vi "读取CODMn数据波形新.vi"() -> ()   [LabVIEW 2016, in "斯坦道CODMn.lvlib"]
uses:
  <vilib>/Utility/miscctls.llb/LVPointTypeDef.ctl
  <userlib>/_OpenG.lib/array/array.llb/Sort 1D Array (I32)__ogtk.vi
  <vilib>/Waveform/WDTFileIO.llb/Read Waveform from File.vi
panel:
  in  "页":i32 format="第%.0f页"
  in  "每页条数":i32=20
  in  "向后按钮":bool
  in  "向前按钮":bool
  in  "数据表":T1
  in  "查看曲线数组":bool[](array[boolean])
  in  "打开波形文件":bool
  in  "簇":cluster{"数据起始时间":timestamp, "数据终止时间":timestamp}
  in  "查询":bool
  in  "当前滴定曲线":bool
  in  "当前温度曲线":bool
  in  "关闭":bool
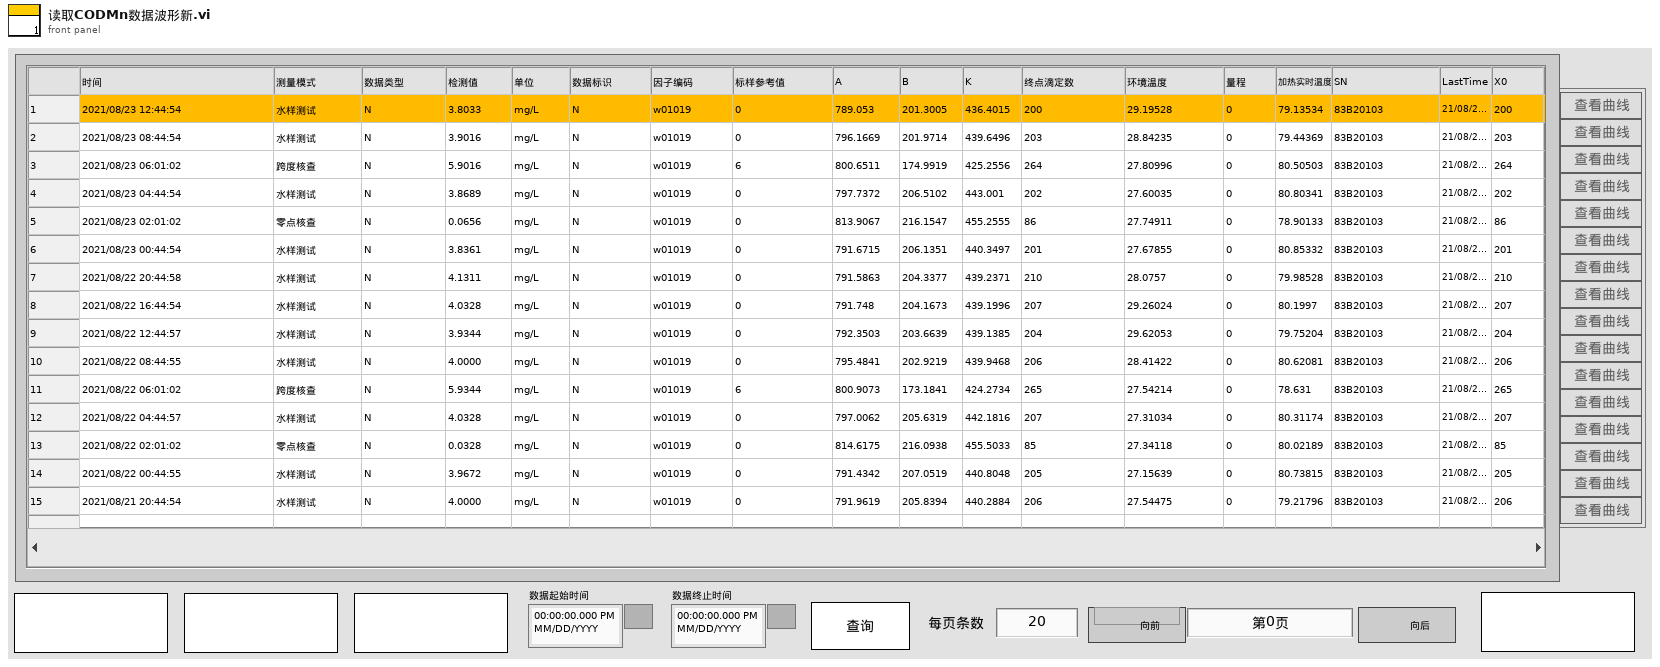
[diagram p1: front panel]
types:
  T1 = typedef "斯坦道CODMn.lvlib/数据查询大列表框.ctl" = i32
  T2 = typedef "LVPointTypeDef.ctl" = cluster{"Horizontal":i16, "Vertical":i16}
  T3 = cluster{timestamp, "seconds since 1Jan1904":timestamp}
  T4 = enum16{"Left Button", "Center Button", "Right Button", "Window Close"}
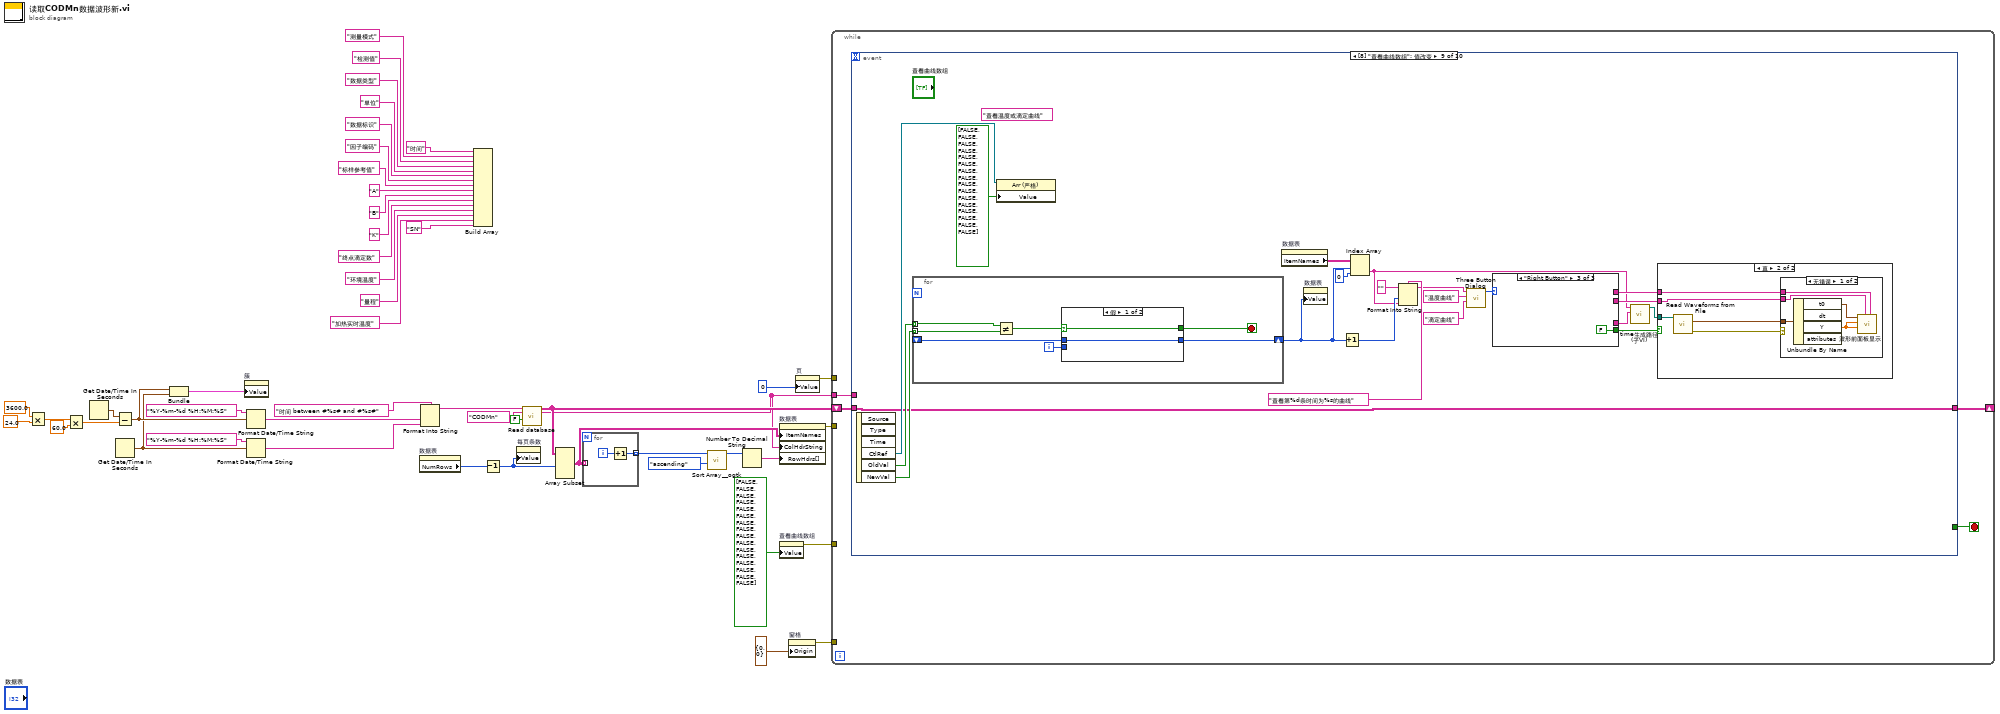
[diagram p0: block diagram]
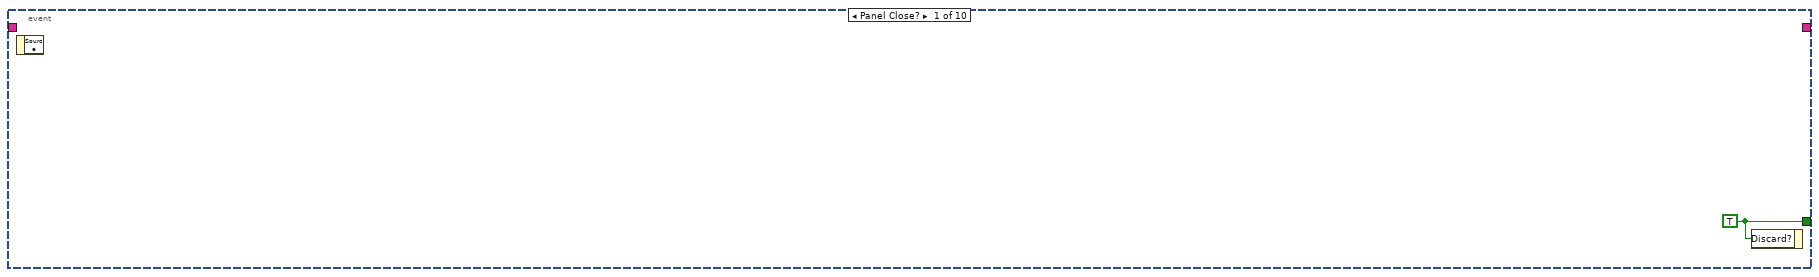
[diagram p2: hidden frame]
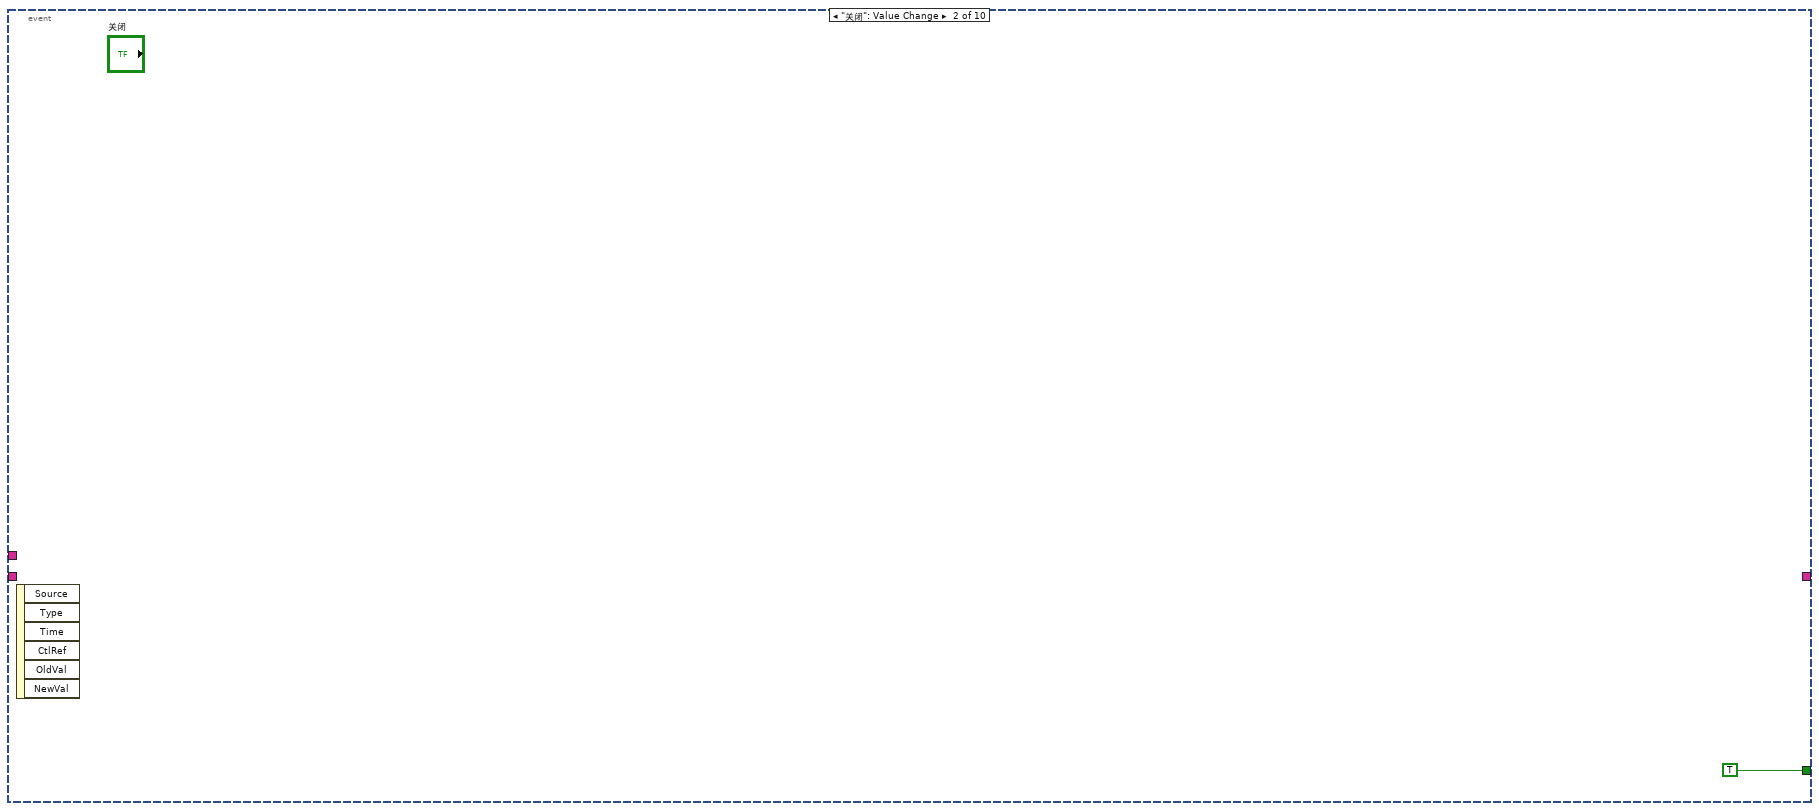
[diagram p3: hidden frame]
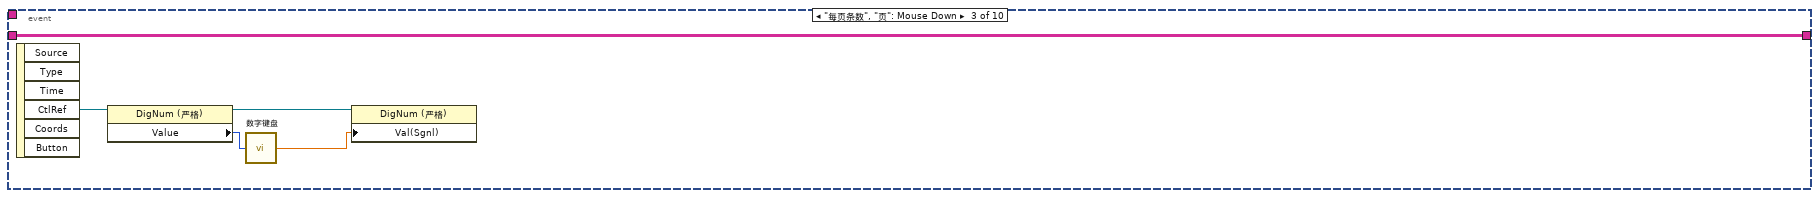
[diagram p4: hidden frame]
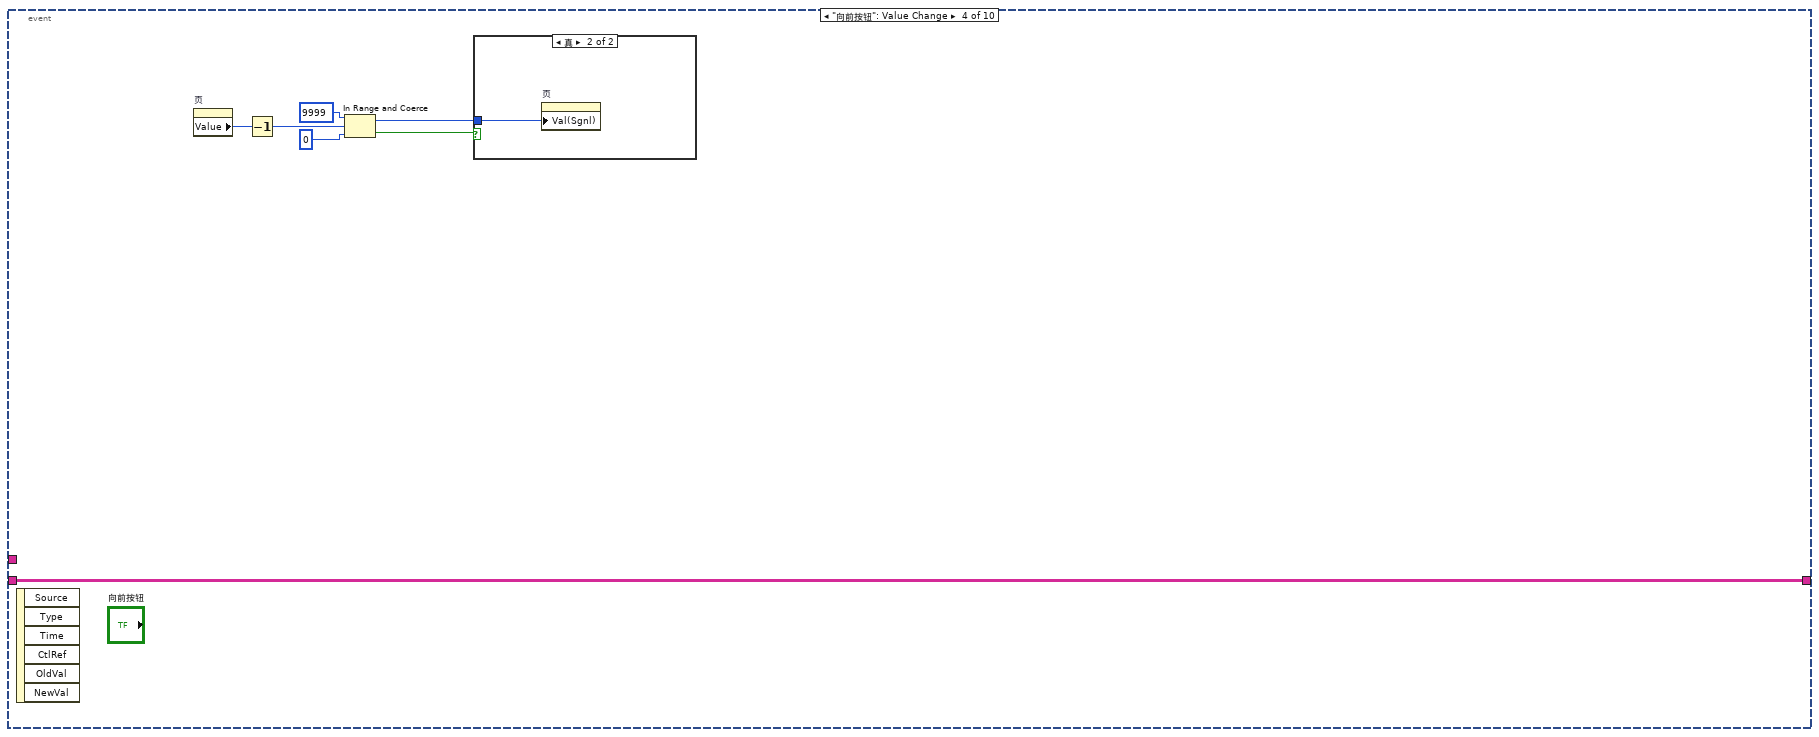
[diagram p5: hidden frame]
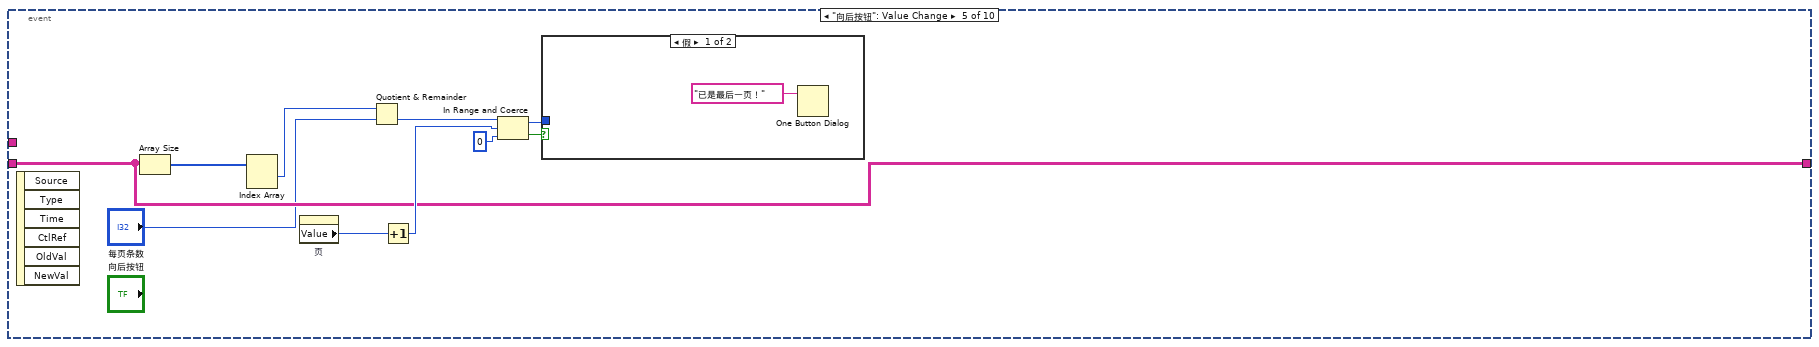
[diagram p7: hidden frame]
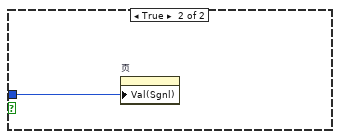
[diagram p8: hidden frame]
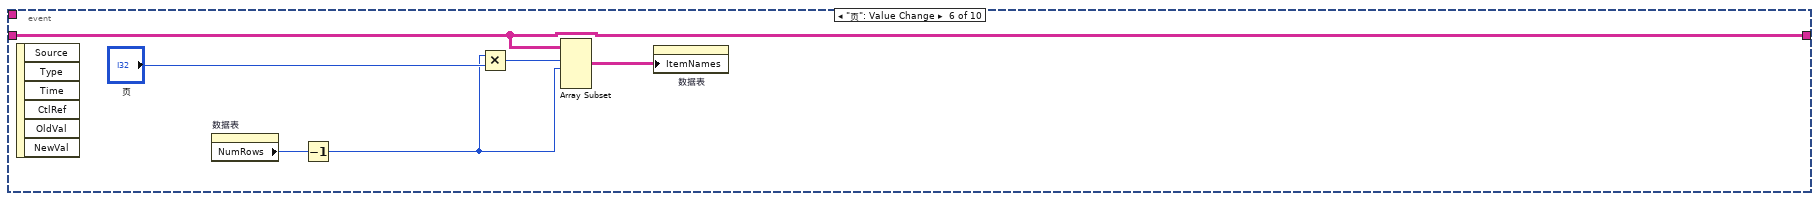
[diagram p9: hidden frame]
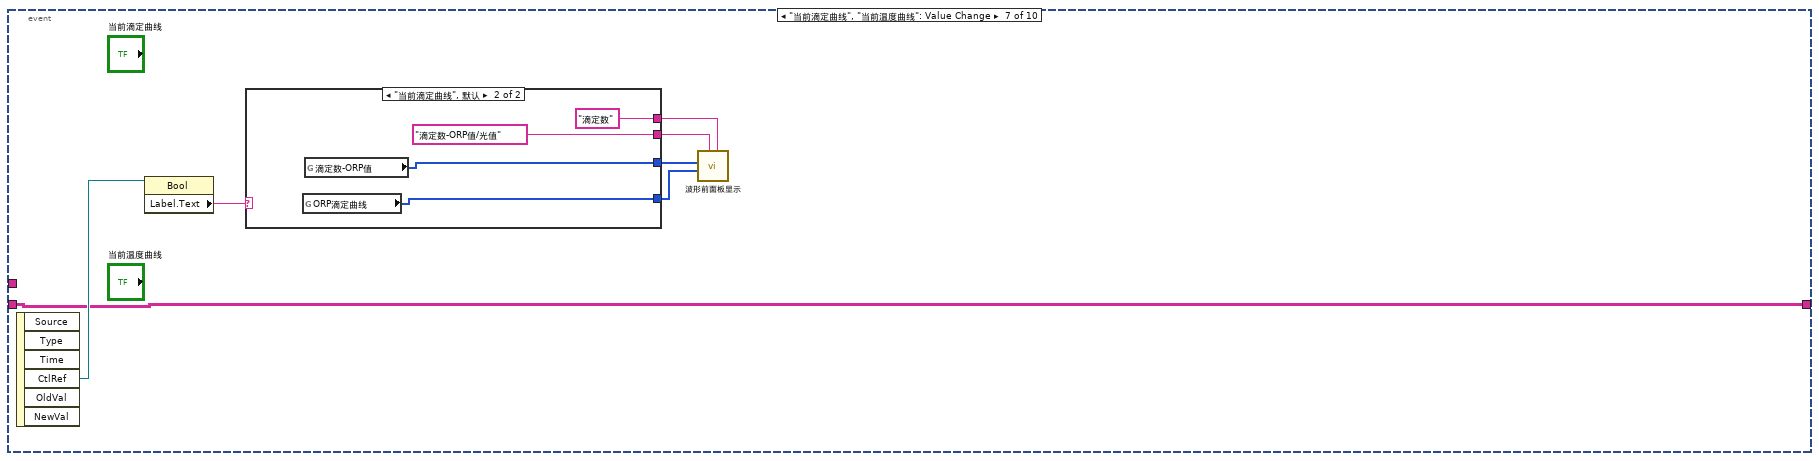
[diagram p10: hidden frame]
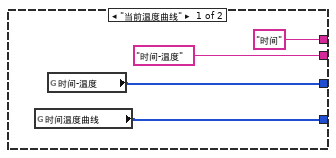
[diagram p11: hidden frame]
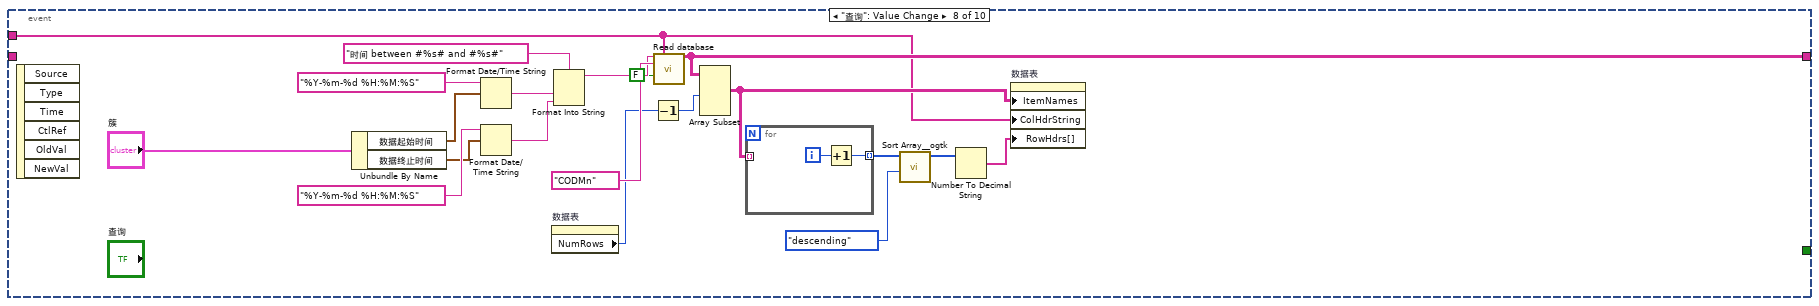
[diagram p12: hidden frame]
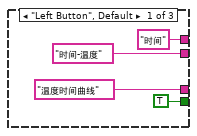
[diagram p14: hidden frame]
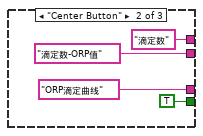
[diagram p15: hidden frame]
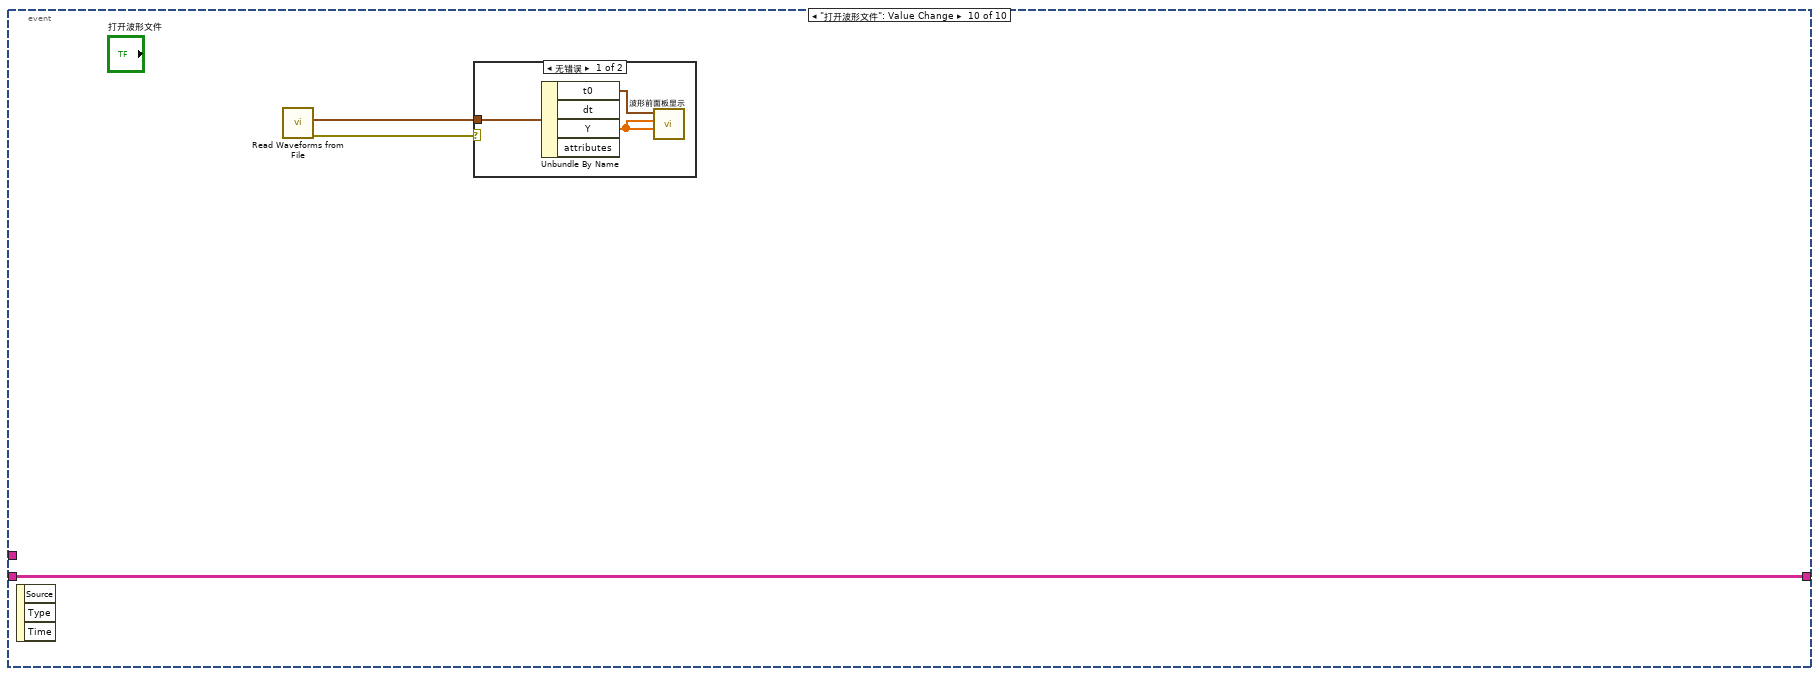
[diagram p18: hidden frame]
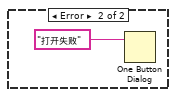
[diagram p19: hidden frame]
diagram:
  n1 = Multiply(x=3600.0, y=24.0) -> (x*y=w46:dbl)
  n2 = Multiply(x=w46, y=60.0) -> (x*y=w44:dbl)
  n3 = Get Date/Time In Seconds() -> (seconds since 1Jan1904=w49:timestamp)
  n4 = Subtract(x=w49, y=w44) -> (x-y=w23:timestamp)
  n5 = Get Date/Time In Seconds() -> (seconds since 1Jan1904=w22:timestamp)
  n6 = Bundle(w23, "seconds since 1Jan1904"=w22) -> (w21:T3)  [unwired: 1 in]
  n7 = property on="簇" class="Clust (严格)"("Value"=w21) -> ()  [unwired: 2 in, 2 out]
  n8 = Format Date/Time String(time format string (%c)="%Y-%m-%d %H:%M:%S" ("时间格式字符串(%c)"), seconds (now)=w23) -> (date/time string=w42:string)  [unwired: 1 in]
  n9 = Format Date/Time String(time format string (%c)="%Y-%m-%d %H:%M:%S" ("时间格式字符串(%c)"), seconds (now)=w22) -> (date/time string=w43:string)  [unwired: 1 in]
  n10 = property on="数据表" class="MCListbox (严格)"() -> ("NumRows"=w33:u32)  [unwired: 2 in, 2 out]
  n11 = Format Into String(format string="时间 between #%s# and #%s#" ("condition"), w42, w43) -> (resulting string=w3:string)  [unwired: 2 in, 1 out]
  n12 = Build Array("时间", "测量模式", "检测值", "数据类型", "单位", "数据标识", "因子编码", "标样参考值", "A", "B", "K", "终点滴定数", "环境温度", "量程", "加热实时温度", "SN") -> ()  [unwired: 1 out]
  n13 = Decrement(x=w33) -> (x-1=w31:u32)
  n14 = property on="每页条数" class="DigNum (严格)"("Value"=w31) -> ()  [unwired: 2 in, 2 out]
  n15 = call "Read database.vi"("condition"=w3, "Table"="CODMn" ("组合框"), "量程筛选"=FALSE) -> ("表格"=w30:string[][], "columns"=w1:string[])  [unwired: 8 in, 3 out]
  n16 = Array Subset(array=w30, length (row)=w31) -> (w32:string[][])  [unwired: 3 in]
  n17 = for {
    tunnel: [w50] -> w38 mode=indexing
    tunnel: w32 -> [_] mode=indexing
    i -> [w51]
    n18 = Increment(x=w51) -> (x+1=w50:i32)
  }
  n19 = call-poly <userlib>:"Sort Array__ogtk.vi"("Order"=enum16{"ascending", "descending"}."ascending", "Array in"=w38) -> ("Sorted Array out"=w36:i32[])  [unwired: 8 in, 1 out]
  n20 = Number To Decimal String(number=w36) -> (decimal integer string=w35:string[])  [unwired: 1 in]
  n21 = property on="数据表" class="MCListbox (严格)"("ItemNames"=w32, "ColHdrString"=w1, "RowHdrs[]"=w35) -> (error out=w34:errorcluster)  [unwired: 2 in, 1 out]
  n22 = property on="查看曲线数组" class="Arr (严格)"("Value"=bool[] [FALSE, FALSE, FALSE, FALSE, FALSE, FALSE, FALSE, FALSE, FALSE, FALSE, FALSE, FALSE, FALSE, FALSE, FALSE, FALSE] ("查看曲线数组")) -> (error out=w24:errorcluster)  [unwired: 2 in, 1 out]
  n23 = property on="窗格" class="Pane"("Origin"=T2 {"Horizontal"=0, "Vertical"=0} ("原点")) -> (error out=w26:errorcluster)  [unwired: 2 in, 1 out]
  n24 = property on="页" class="DigNum (严格)"("Value"=0 ("页")) -> (error out=w28:errorcluster)  [unwired: 2 in, 1 out]
  n25 = while {
    tunnel: w34 -> [_]
    shift-right: [w53] -> _
    shift-left: w30 -> [w54]
    tunnel: w28 -> [_]
    tunnel: w26 -> [_]
    tunnel: w24 -> [_]
    tunnel: w1 -> [w52]
    stop <- w55 stop-if-true
    n26 = event shown="[8] \"查看曲线数组\": 值改变" {
      selector: _ -> [_ _ _ _ _ _ _ _ _ _]
      dyn-events: _ -> [_ _ _ _ _ _ _ _ _ _]
      timeout: _ -> [_ _ _ _ _ _ _ _ _ _]
      tunnel: [w56 TRUE ("Discard?") _ _ _ _ _ _ _ _] -> w55
      tunnel: w54 -> [_ _ w58 w63 w75 w83 w89 _ w130 w177]
      tunnel: [_ _ w58 w63 w75 w83 w89 w107 w130 w177] -> w53
      tunnel: w52 -> [_ _ _ _ _ _ _ w105 _ _]
      event Panel Close? {
        w56 = TRUE ("Discard?")
        n27 = event-data() -> ()  [unwired: 1 in, 1 out]
        n28 = event-data("Discard?"=w56) -> ()  [unwired: 1 in, 1 out]
      }
      event "关闭": Value Change {
        n29 = event-data() -> ()  [unwired: 1 in, 6 out]
      }
      event "每页条数", "页": Mouse Down {
        n30 = event-data() -> ("CtlRef"=w62:refnum<vi>)  [unwired: 1 in, 5 out]
        n31 = property class="DigNum (严格)"(reference=w62) -> (reference out=w60:refnum<vi>, "Value"=w61:i32)  [unwired: 1 in, 1 out]
        n32 = call "数字键盘.vi"("OldNumber"=w61) -> ("NewNumber"=w59:sgl)
        n33 = property class="DigNum (严格)"(reference=w60, "Val(Sgnl)"=w59) -> ()  [unwired: 1 in, 2 out]
      }
      event "向前按钮": Value Change {
        n34 = event-data() -> ()  [unwired: 1 in, 6 out]
        n35 = property on="页" class="DigNum (严格)"() -> ("Value"=w64:i32)  [unwired: 2 in, 2 out]
        n36 = Decrement(x=w64) -> (x-1=w69:i32)
        n37 = In Range and Coerce(upper limit=9999 ("上限"), x=w69, lower limit=0 ("下限")) -> (coerced(x)=w66:i32, In Range?=w65:bool)
        n38 = case shown="真" w65 {
          tunnel: w66 -> [_ w70]
          frame False {
          }
          frame True {
            n39 = property on="页" class="DigNum (严格)"("Val(Sgnl)"=w70) -> ()  [unwired: 2 in, 2 out]
          }
        }
      }
      event "向后按钮": Value Change {
        n40 = event-data() -> ()  [unwired: 1 in, 6 out]
        n41 = Array Size(array=w75) -> (size(s)=w74:i32[])
        n42 = Index Array(array=w74) -> (element #1=w73:i32)  [unwired: 2 in, 1 out]
        n43 = property on="页" class="DigNum (严格)"() -> ("Value"=w76:i32)  [unwired: 2 in, 2 out]
        n44 = Quotient & Remainder(x=w73, y="每页条数") -> (floor(x/y)=w71:i32)  [unwired: 1 out]
        n45 = Increment(x=w76) -> (x+1=w80:i32)
        n46 = In Range and Coerce(upper limit=w71, x=w80, lower limit=0 ("下限")) -> (coerced(x)=w78:i32, In Range?=w77:bool)
        n47 = case shown="假" w77 {
          tunnel: w78 -> [_ w82]
          frame False {
            n48 = One Button Dialog(message="已是最后一页！" ("消息")) -> ()  [unwired: 1 in, 1 out]
          }
          frame True {
            n49 = property on="页" class="DigNum (严格)"("Val(Sgnl)"=w82) -> ()  [unwired: 2 in, 2 out]
          }
        }
      }
      event "页": Value Change {
        n50 = event-data() -> ()  [unwired: 1 in, 6 out]
        n51 = property on="数据表" class="MCListbox (严格)"() -> ("NumRows"=w87:u32)  [unwired: 2 in, 2 out]
        n52 = Decrement(x=w87) -> (x-1=w85:u32)
        n53 = Multiply(x=w85, y="页") -> (x*y=w86:u32)
        n54 = Array Subset(array=w83, index (row)=w86, length (row)=w85) -> (w84:string[][])  [unwired: 2 in]
        n55 = property on="数据表" class="MCListbox (严格)"("ItemNames"=w84) -> ()  [unwired: 2 in, 2 out]
      }
      event "当前滴定曲线", "当前温度曲线": Value Change {
        n56 = event-data() -> ("CtlRef"=w93:refnum<vi>)  [unwired: 1 in, 5 out]
        n57 = property class="Bool"(reference=w93) -> ("Label.Text"=w92:string)  [unwired: 1 in, 2 out]
        n58 = case shown="\"当前滴定曲线\", 默认" w92 {
          tunnel: [w96 w100] -> w95
          tunnel: [w97 w101] -> w94
          tunnel: ["时间-温度" ("标题.文本") "滴定数-ORP值/光值" ("标题.文本")] -> w91
          tunnel: ["时间" ("X标尺.名称标签.文本") "滴定数" ("X标尺.名称标签.文本")] -> w90
          frame "当前温度曲线" {
            n59 = global read "COD内部交互全局.vi" "时间温度曲线"() -> (w96:u16[])
            n60 = global read "COD内部交互全局.vi" "时间-温度"() -> (w97:u16[])
          }
          frame "当前滴定曲线", Default {
            n61 = global read "COD内部交互全局.vi" "ORP滴定曲线"() -> (w100:u16[])
            n62 = global read "COD内部交互全局.vi" "滴定数-ORP值"() -> (w101:u16[])
          }
        }
        n63 = call "波形前面板显示.vi"("X标尺.名称标签.文本"=w90, "标题.文本"=w91, "ORP滴定曲线"=w95, "滴定数-ORP值"=w94) -> ()  [unwired: 8 in]
      }
      event "查询": Value Change {
        n64 = event-data() -> ()  [unwired: 1 in, 6 out]
        n65 = Unbundle By Name("簇") -> ("数据起始时间"=w116:timestamp, "数据终止时间"=w115:timestamp)
        n66 = Format Date/Time String(time format string (%c)="%Y-%m-%d %H:%M:%S" ("时间格式字符串(%c)"), seconds (now)=w116) -> (date/time string=w120:string)  [unwired: 1 in]
        n67 = Format Date/Time String(time format string (%c)="%Y-%m-%d %H:%M:%S" ("时间格式字符串(%c)"), seconds (now)=w115) -> (date/time string=w121:string)  [unwired: 1 in]
        n68 = property on="数据表" class="MCListbox (严格)"() -> ("NumRows"=w109:u32)  [unwired: 2 in, 2 out]
        n69 = Format Into String(format string="时间 between #%s# and #%s#" ("condition"), w120, w121) -> (resulting string=w106:string)  [unwired: 2 in, 1 out]
        n70 = Decrement(x=w109) -> (x-1=w110:u32)
        n71 = call "Read database.vi"("condition"=w106, "显示项"=w105, "Table"="CODMn" ("组合框"), "量程筛选"=FALSE) -> ("表格"=w107:string[][])  [unwired: 7 in, 4 out]
        n72 = Array Subset(array=w107, length (row)=w110) -> (w108:string[][])  [unwired: 3 in]
        n73 = for {
          tunnel: [w124] -> w114 mode=indexing
          tunnel: w108 -> [_] mode=indexing
          i -> [w125]
          n74 = Increment(x=w125) -> (x+1=w124:i32)
        }
        n75 = call-poly <userlib>:"Sort Array__ogtk.vi"("Order"=enum16{"ascending", "descending"}."descending", "Array in"=w114) -> ("Sorted Array out"=w112:i32[])  [unwired: 8 in, 1 out]
        n76 = Number To Decimal String(number=w112) -> (decimal integer string=w111:string[])  [unwired: 1 in]
        n77 = property on="数据表" class="MCListbox (严格)"("ItemNames"=w108, "ColHdrString"=w105, "RowHdrs[]"=w111) -> ()  [unwired: 2 in, 2 out]
      }
      event "查看曲线数组": Value Change {
        (unwired) "查看温度或滴定曲线" ("message")
        n78 = event-data() -> ("CtlRef"=w136:refnum<vi>, "OldVal"=w138:bool[], "NewVal"=w137:bool[])  [unwired: 1 in, 3 out]
        n79 = for {
          tunnel: w138 -> [w153] mode=indexing
          tunnel: w137 -> [w152] mode=indexing
          shift-right: [w149] -> w129
          shift-left: _ -> [w148]
          i -> [w150]
          stop <- w147 stop-if-true
          n80 = Not Equal?(x=w153, y=w152) -> (x != y?=w151:bool)
          n81 = case shown="假" w151 {
            selector: w151 -> [w155 w156]
            tunnel: w150 -> [_ w157]
            tunnel: [w154 w157] -> w149
            tunnel: [w155 w156] -> w147
            tunnel: w148 -> [w154 _]
            frame False {
            }
            frame True {
            }
          }
        }
        n82 = property class="Arr (严格)"(reference=w136, "Value"=bool[] [FALSE, FALSE, FALSE, FALSE, FALSE, FALSE, FALSE, FALSE, FALSE, FALSE, FALSE, FALSE, FALSE, FALSE, FALSE, FALSE] ("查看曲线数组")) -> ()  [unwired: 1 in, 2 out]
        n83 = property on="数据表" class="MCListbox (严格)"() -> ("ItemNames"=w126:string[][])  [unwired: 2 in, 2 out]
        n84 = property on="数据表" class="MCListbox (严格)"("Value"=w129) -> ()  [unwired: 2 in, 2 out]
        n85 = Increment(x=w129) -> (x+1=w131:i32)
        n86 = Index Array(array=w126, index (row)=w129, index (col)=0 ("长度")) -> (element=w127:string)
        n87 = Format Into String(format string="查看第%d条时间为%s的曲线" ("格式字符串"), initial string="" ("初始字符串"), w131, w127) -> (resulting string=w132:string)  [unwired: 1 in, 1 out]
        n88 = call <vilib>:"Three Button Dialog.vi"("Center Button Text (\"No\")"="滴定曲线" ("Center Button Text (\"No\")"), "Left Button Text (\"Yes\")"="温度曲线" ("Left Button Text (\"Yes\")"), "message"=w132) -> ("Which Button?"=w140:T4)  [unwired: 8 in]
        n89 = case shown="\"Right Button\"" w140 {
          tunnel: ["温度时间曲线" ("名称或相对路径") "ORP滴定曲线" ("名称或相对路径") _] -> w145
          tunnel: ["时间-温度" ("标题.文本") "滴定数-ORP值" ("标题.文本") _] -> w144
          tunnel: ["时间" ("X标尺.名称标签.文本") "滴定数" ("X标尺.名称标签.文本") _] -> w143
          tunnel: [TRUE TRUE FALSE] -> w139
          frame "Left Button", Default {
          }
          frame "Center Button" {
          }
          frame "Right Button" {
          }
        }
        n90 = call "time生成路径 (子VI).vi"("名称或相对路径"=w145, "时间"=w127) -> ("appended path"=w146:path)  [unwired: 9 in]
        n91 = case shown="真" w139 {
          tunnel: w146 -> [_ w169]
          tunnel: w144 -> [_ w168]
          tunnel: w143 -> [_ w167]
          frame False {
          }
          frame True {
            n92 = call-poly <vilib>:"Read Waveforms from File.vi"("file path (dialog if empty)"=w169) -> ("error out"=w171:errorcluster, "first waveform in record"=w170:waveform(dbl))  [unwired: 5 in, 2 out]
            n93 = case shown="无错误" w171 {
              tunnel: w170 -> [w176 _]
              tunnel: w168 -> [w173 _]
              tunnel: w167 -> [w172 _]
              frame No Error {
                n94 = Unbundle By Name(w176) -> ("t0"=w175:timestamp, "Y"=w174:dbl[])  [unwired: 2 out]
                n95 = call "波形前面板显示.vi"("X标尺.名称标签.文本"=w172, "标题.文本"=w173, "ORP滴定曲线"=w174, "滴定数-ORP值"=w174, "波形时间"=w175) -> ()  [unwired: 7 in]
              }
              frame Error {
              }
            }
          }
        }
      }
      event "打开波形文件": Value Change {
        n96 = event-data() -> ()  [unwired: 1 in, 3 out]
        n97 = call-poly <vilib>:"Read Waveforms from File.vi"() -> ("error out"=w179:errorcluster, "first waveform in record"=w178:waveform(dbl))  [unwired: 6 in, 2 out]
        n98 = case shown="无错误" w179 {
          tunnel: w178 -> [w182 _]
          frame No Error {
            n99 = Unbundle By Name(w182) -> ("t0"=w181:timestamp, "Y"=w180:dbl[])  [unwired: 2 out]
            n100 = call "波形前面板显示.vi"("ORP滴定曲线"=w180, "滴定数-ORP值"=w180, "波形时间"=w181) -> ()  [unwired: 9 in]
          }
          frame Error {
            n101 = One Button Dialog(message="打开失败" ("消息")) -> ()  [unwired: 1 in, 1 out]
          }
        }
      }
    }
  }
